vi "process_display.vi"() -> ()   [LabVIEW 2011, in "Fiberscope_library.lvlib"]
uses:
  Fiberscope_library.lvlib
  typedefs/control_process_state_cluster.ctl
  typedefs/control_process_state_enum.ctl
  typedefs/element_images_cluster.ctl
  typedefs/feedback_to_watchdog.ctl
  typedefs/feedback_from_process_enum.ctl
  typedefs/image_size_I32.ctl
  <vilib>/Analysis/NI_AALBase.lvlib
panel:
  out "Ch1 Min":u16
  out "Ch1 Max":u16
  in  "Ch1 Software gain":dbl=1.0 min=0.5 max=2.0 step=0.1
  in  "Ch1 Full range":bool
  in  "Ch1 Optimize":bool
  in  "Ch1 Color":T1(radio)
  out "Ch1 Histogram":T2(graph)
  out "Channel 1":u16[][](graph)
  in  "Ch0 Software gain":dbl=1.0 min=0.5 max=2.0 step=0.1
  out "Ch0 Histogram":T2(graph)
  in  "Ch0 Color":T1(radio)
  out "Ch0 Min":u16
  out "Ch0 Max":u16
  in  "Ch0 Full range":bool
  out "Channel 0":u16[][](graph)
  in  "Ch0 Optimize":bool
  out "Local exit":bool
  out "error out":errorcluster
  in  "error in":errorcluster
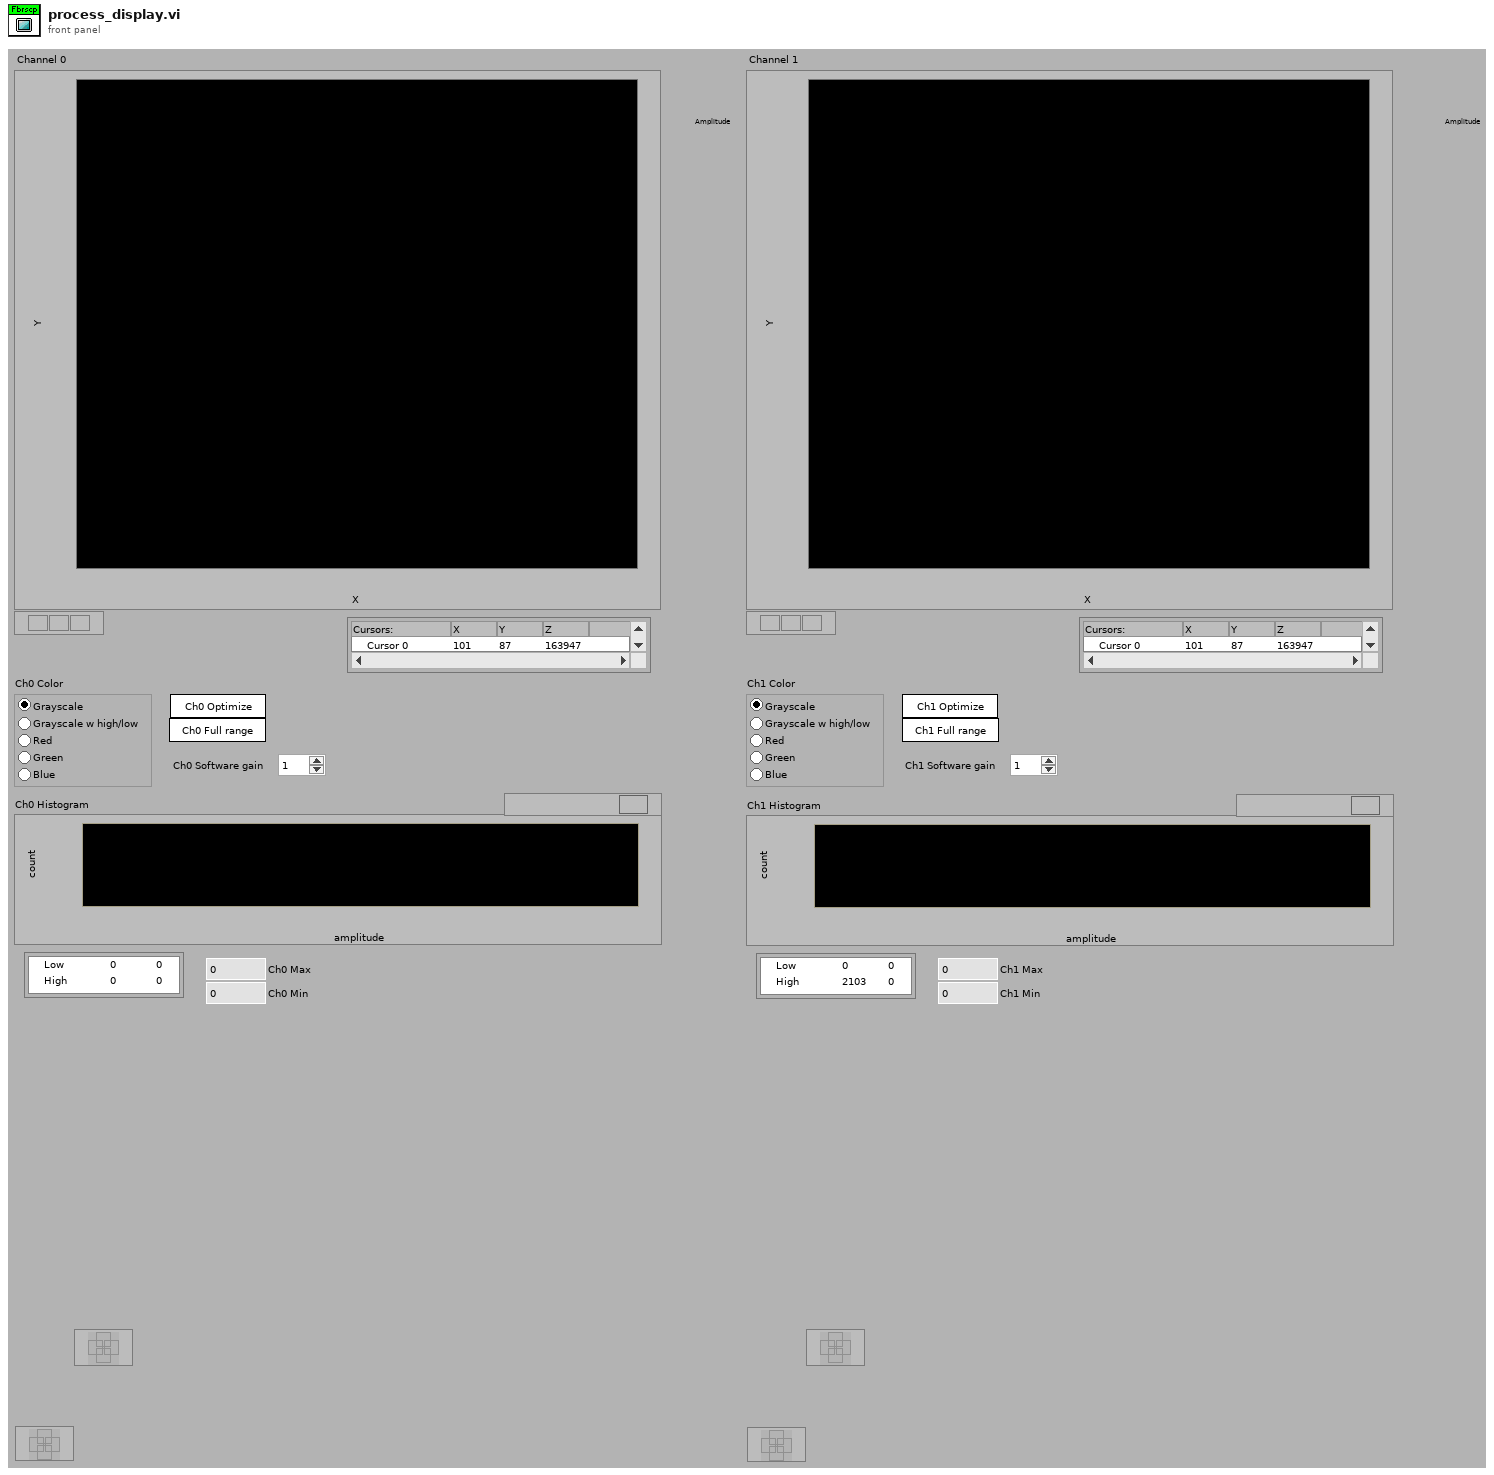
[diagram p1: front panel]
types:
  T1 = enum32{"Grayscale", "Grayscale w high/low", "Red", "Green", "Blue"}
  T2 = cluster{"X Values":dbl[], "Histogram: h(x)":i32[]}
  T3 = typedef "Fiberscope_library.lvlib/feedback_to_watchdog.ctl" = cluster{"Feedback_from_process_enum":T4, "Process_name":string}
  T4 = typedef "Fiberscope_library.lvlib/feedback_from_process_enum.ctl" = enum16{"Has_initialised", "Changed_parameters", "Has_started", "Has_stopped", "Has_quitted", "Is_running", "Has_finished", "Custom"}
  T5 = typedef "Fiberscope_library.lvlib/element_images_cluster.ctl" = cluster{"Images_array":dbl[][][], "#channels":i32, "Last element?":bool}
  T6 = typedef "Fiberscope_library.lvlib/control_process_state_cluster.ctl" = cluster{"Control_process_state_enum":T7, "variant":variant}
  T7 = typedef "Fiberscope_library.lvlib/control_process_state_enum.ctl" = enum16{"Init", "Quit", "Start", "Stop", "Change_parameters", "Running", "Finish", "Custom"}
  T8 = typedef "LVCursorListTypeDef.ctl" = cluster{"Name":string, "Color":u32, "Style":u8, "Point Style":u8, "Name Visible":bool, "Allow Drag":bool, "Cursor Mode":u32, "Plot":i32, "Index":i32, "Position":cluster{"X":dbl, "Y":dbl}, "X Scale":u32, "Y Scale":u32, "Watch Plots":i32[], "Watch All Plots":bool, "Plot Area":i32, "Label Offset":cluster{"X":dbl, "Y":dbl}}[]
  T9 = cluster{"Name":string, "Color":u32, "Style":u8, "Point Style":u8, "Name Visible":bool, "Allow Drag":bool, "Cursor Mode":u32, "Plot":i32, "Index":i32, "Position":cluster{"X":dbl, "Y":dbl}, "X Scale":u32, "Y Scale":u32, "Watch Plots":i32[], "Watch All Plots":bool, "Plot Area":i32, "Label Offset":cluster{"X":dbl, "Y":dbl}}
  T10 = cluster{"Name":string, "Color":u32, "Style":u8, "Point Style":u8, "Name Visible":bool, "Allow Drag":bool, "Cursor Mode":u32, "Plot":i32, "Index":i32, "Position":cluster{"X":dbl, "Y":dbl}, "X Scale":u32, "Y Scale":u32, "Watch Plots":i32[], "Watch All Plots":bool, "Plot Area":i32, "Label Offset":cluster{"X":dbl, "Y":dbl}}[]
  T11 = typedef "Fiberscope_library.lvlib/image_size_I32.ctl" = i32
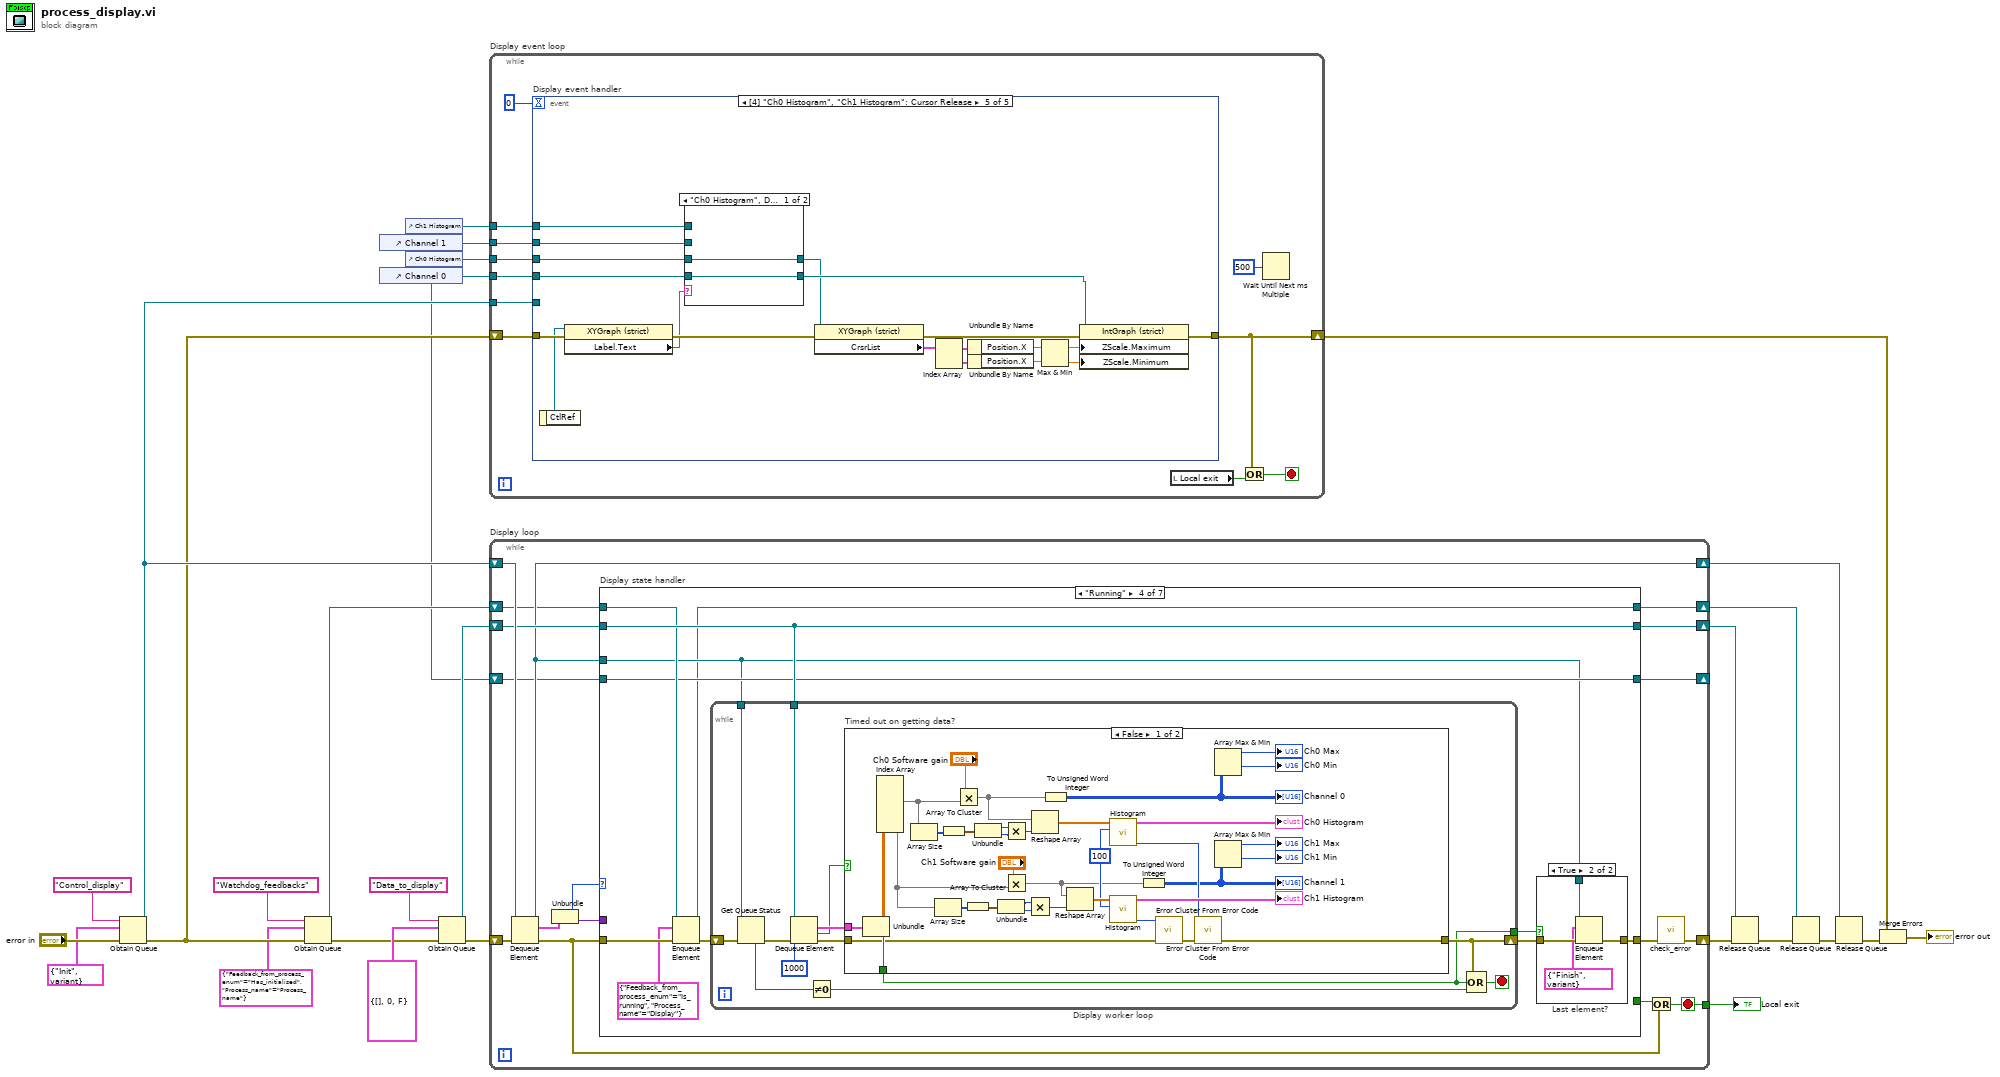
[diagram p0: block diagram]
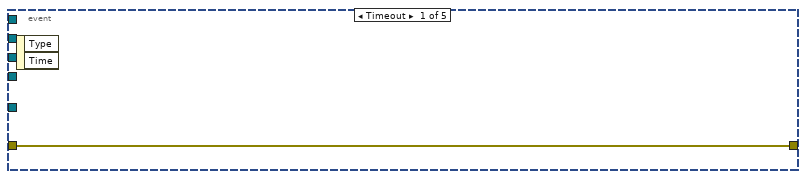
[diagram p2: hidden frame]
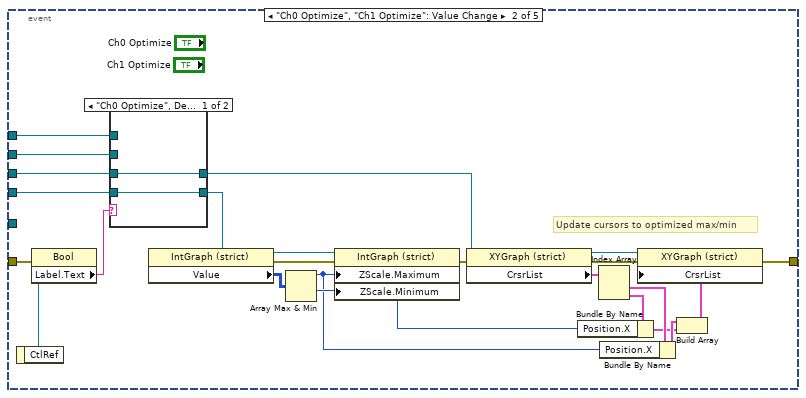
[diagram p3: hidden frame]
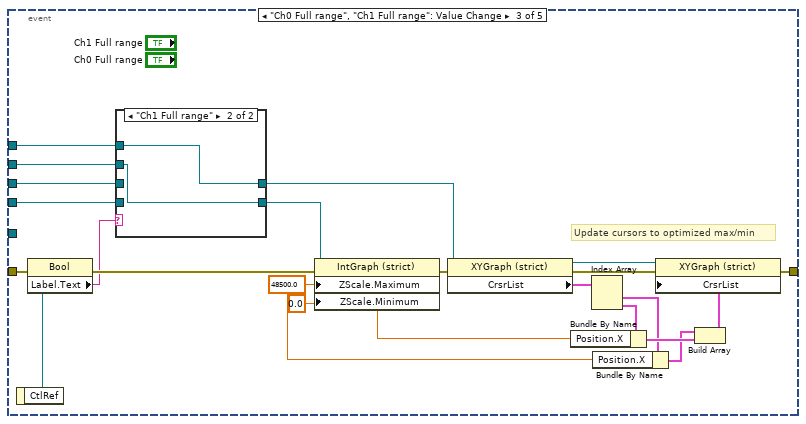
[diagram p5: hidden frame]
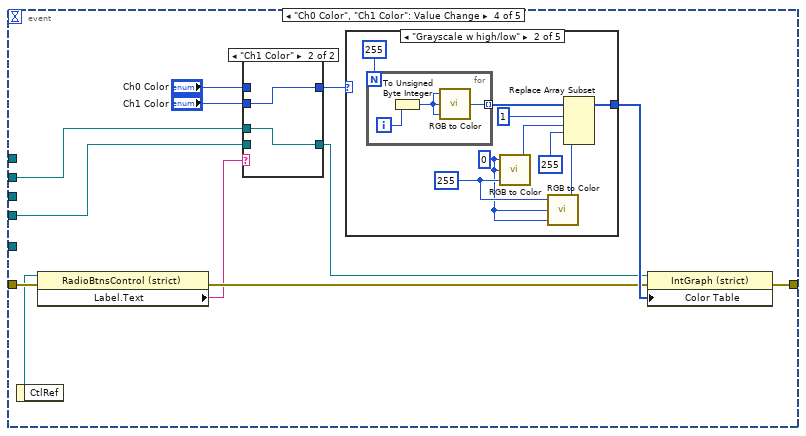
[diagram p7: hidden frame]
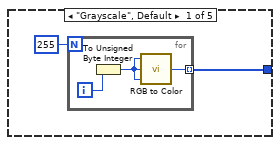
[diagram p9: hidden frame]
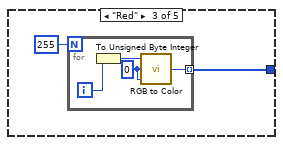
[diagram p10: hidden frame]
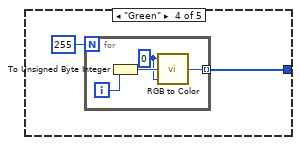
[diagram p11: hidden frame]
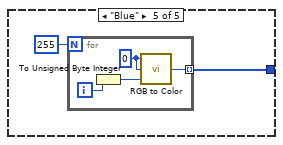
[diagram p12: hidden frame]
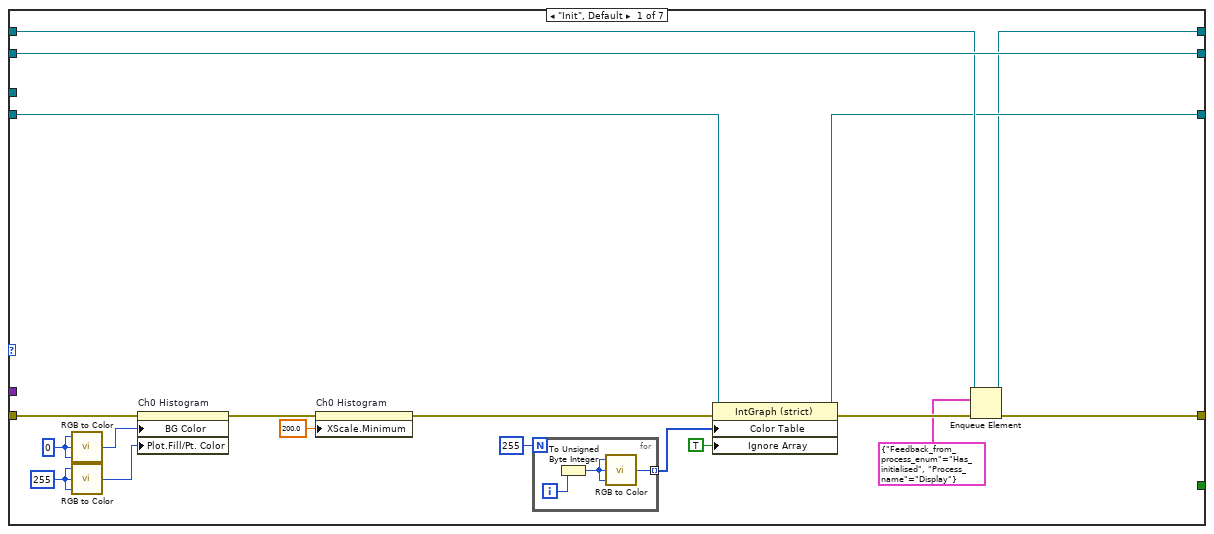
[diagram p14: hidden frame]
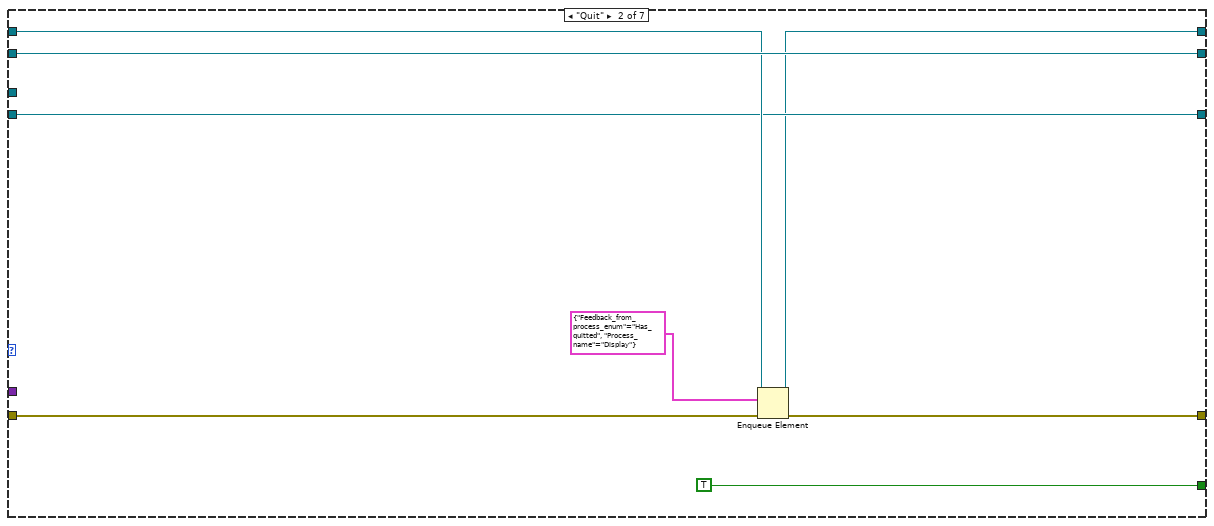
[diagram p15: hidden frame]
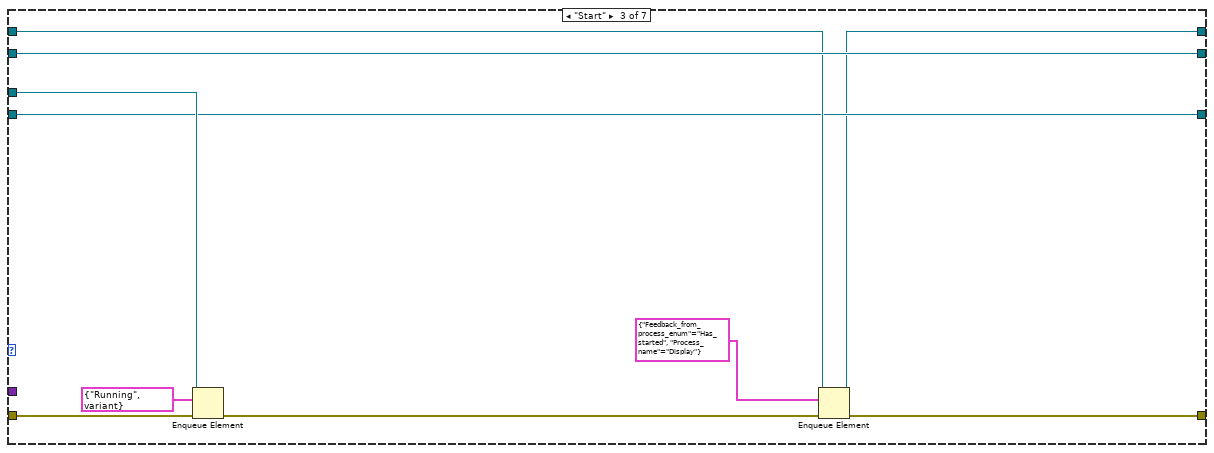
[diagram p16: hidden frame]
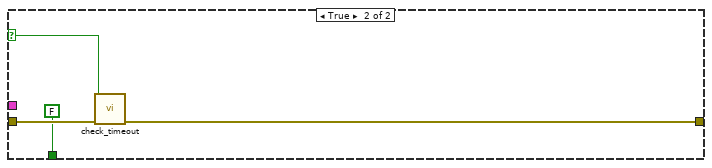
[diagram p18: hidden frame]
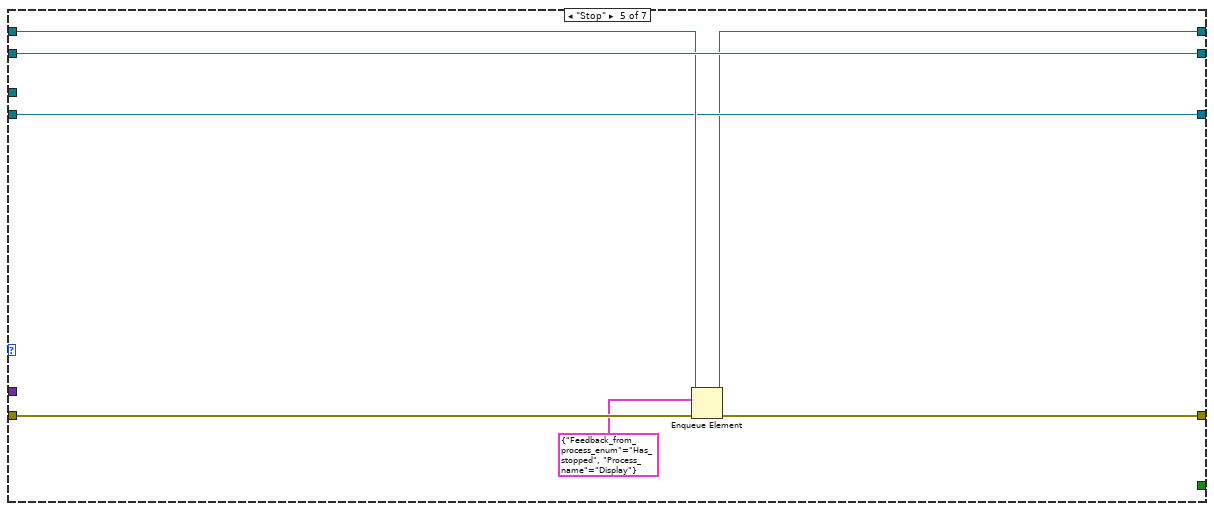
[diagram p19: hidden frame]
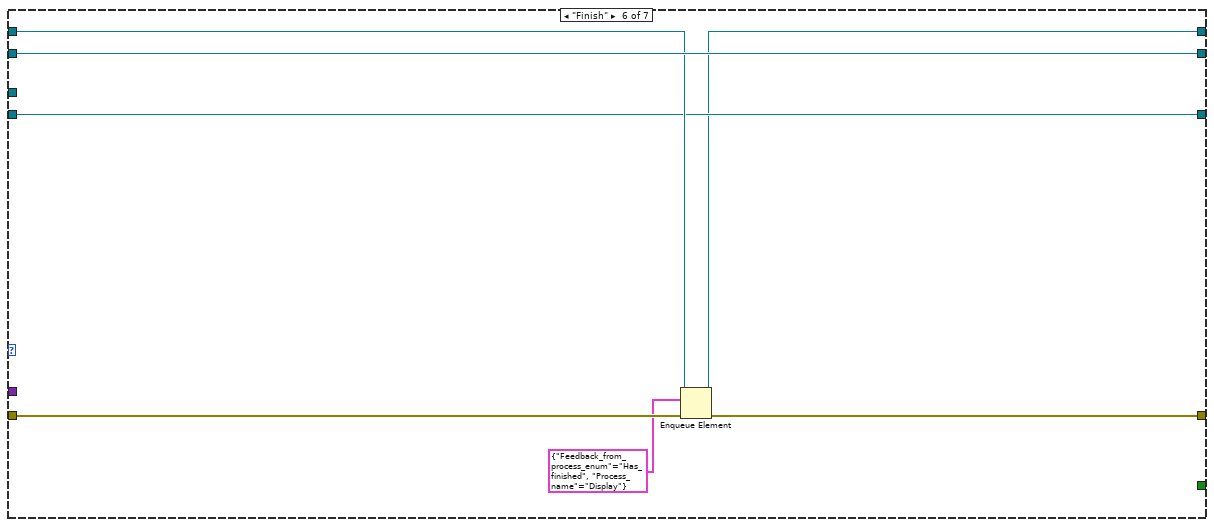
[diagram p20: hidden frame]
diagram:
  n1 = Obtain Queue(name (unnamed)="Control_display", element data type=T6 {"Control_process_state_enum"=enum."Init", "variant"=variant} ("Control_process_state_cluster"), error in (no error)="error in") -> (queue out=w16:refnum<queue>, error out=w11:errorcluster)  [unwired: 2 in, 1 out]
  n2 = Obtain Queue(name (unnamed)="Watchdog_feedbacks", element data type=T3 {"Feedback_from_process_enum"=enum."Has_initialised", "Process_name"="Process_name"}, error in (no error)=w11) -> (queue out=w9:refnum<queue>, error out=w10:errorcluster)  [unwired: 2 in, 1 out]
  n3 = control-ref of="Channel 1"() -> (w2:refnum<vi>)
  n4 = control-ref of="Channel 0"() -> (w5:refnum<vi>)
  n5 = control-ref of="Ch1 Histogram"() -> (w1:refnum<vi>)
  n6 = control-ref of="Ch0 Histogram"() -> (w4:refnum<vi>)
  n7 = Obtain Queue(name (unnamed)="Data_to_display", element data type=T5 {"Images_array"=[], "#channels"=0, "Last element?"=FALSE} ("Image out"), error in (no error)=w10) -> (queue out=w21:refnum<queue>, error out=w23:errorcluster)  [unwired: 2 in, 1 out]
  n8 = while "Display event loop" {
    tunnel: w16 -> [w37]
    shift-right: [w32] -> w14
    shift-left: w11 -> [w36]
    tunnel: w4 -> [w30]
    tunnel: w5 -> [w31]
    tunnel: w2 -> [w29]
    tunnel: w1 -> [w28]
    stop <- w33 stop-if-true
    n9 = event "Display event handler" shown="[4] \"Ch0 Histogram\", \"Ch1 Histogram\": Cursor Release" {
      selector: _ -> [_ _ _ _ _]
      dyn-events: _ -> [_ _ _ _ _]
      timeout: 0 -> [_ _ _ _ _]
      tunnel: w37 -> [_ _ _ _ _]
      tunnel: w36 -> [w39 w40 w77 w103 w148]
      tunnel: [w39 w60 w80 w105 w161] -> w32
      tunnel: w31 -> [_ w45 w71 w97 w154]
      tunnel: w30 -> [_ w46 w72 _ w153]
      tunnel: w29 -> [_ w47 w73 w96 w152]
      tunnel: w28 -> [_ w48 w74 _ w151]
      event Timeout {
        n10 = event-data() -> ()  [unwired: 1 in, 2 out]
      }
      event "Ch0 Optimize", "Ch1 Optimize": Value Change {
        # "Update cursors to optimized max/min"
        n11 = event-data() -> ("CtlRef"=w42:refnum<vi>)  [unwired: 1 in]
        n12 = property class="Bool"(reference=w42, error in=w40) -> ("Label.Text"=w41:string)  [unwired: 2 out]
        n13 = case shown="\"Ch0 Optimize\", Default" w41 {
          tunnel: w48 -> [_ w66]
          tunnel: w47 -> [_ w67]
          tunnel: w46 -> [w64 _]
          tunnel: w45 -> [w65 _]
          tunnel: [w65 w67] -> w44
          tunnel: [w64 w66] -> w43
          frame "Ch0 Optimize", Default {
          }
          frame "Ch1 Optimize" {
          }
        }
        n14 = property class="IntGraph (strict)"(reference=w44) -> (reference out=w61:refnum<vi>, error out=w63:errorcluster, "Value"=w62:u16[][])  [unwired: 1 in]
        n15 = Array Max & Min(array=w62) -> (max value=w52:u16, min value=w53:u16)  [unwired: 2 out]
        n16 = property class="IntGraph (strict)"(reference=w61, error in=w63, "ZScale.Maximum"=w52, "ZScale.Minimum"=w53) -> (error out=w59:errorcluster)  [unwired: 1 out]
        n17 = property class="XYGraph (strict)"(reference=w43, error in=w59) -> (reference out=w57:refnum<vi>, error out=w58:errorcluster, "CrsrList"=w56:T8)
        n18 = Index Array(array=w56) -> (element #1=w55:T9, element #2=w54:T9)  [unwired: 2 in]
        n19 = Bundle By Name(cluster=w54, "Position.X"=w53) -> (w50:T9)
        n20 = Bundle By Name(cluster=w55, "Position.X"=w52) -> (w51:T9)
        n21 = Build Array(w51, w50) -> (w49:T10)
        n22 = property class="XYGraph (strict)"(reference=w57, error in=w58, "CrsrList"=w49) -> (error out=w60:errorcluster)  [unwired: 1 out]
      }
      event "Ch0 Full range", "Ch1 Full range": Value Change {
        w79 = 0.0 ("Z Scale.Range:Minimum")
        w78 = 48500.0 ("Z Scale.Range:Maximum")
        # "Update cursors to optimized max/min"
        n23 = event-data() -> ("CtlRef"=w75:refnum<vi>)  [unwired: 1 in]
        n24 = property class="Bool"(reference=w75, error in=w77) -> (error out=w76:errorcluster, "Label.Text"=w70:string)  [unwired: 1 out]
        n25 = case shown="\"Ch1 Full range\"" w70 {
          tunnel: w74 -> [_ w92]
          tunnel: w73 -> [_ w93]
          tunnel: w72 -> [w90 _]
          tunnel: w71 -> [w91 _]
          tunnel: [w91 w93] -> w69
          tunnel: [w90 w92] -> w68
          frame "Ch0 Full range", Default {
          }
          frame "Ch1 Full range" {
          }
        }
        n26 = property class="IntGraph (strict)"(reference=w69, error in=w76, "ZScale.Maximum"=w78, "ZScale.Minimum"=w79) -> (error out=w81:errorcluster)  [unwired: 1 out]
        n27 = property class="XYGraph (strict)"(reference=w68, error in=w81) -> (reference out=w83:refnum<vi>, error out=w82:errorcluster, "CrsrList"=w84:T8)
        n28 = Index Array(array=w84) -> (element #1=w85:T9, element #2=w86:T9)  [unwired: 2 in]
        n29 = Bundle By Name(cluster=w86, "Position.X"=w79) -> (w88:T9)
        n30 = Bundle By Name(cluster=w85, "Position.X"=w78) -> (w87:T9)
        n31 = Build Array(w87, w88) -> (w89:T10)
        n32 = property class="XYGraph (strict)"(reference=w83, error in=w82, "CrsrList"=w89) -> (error out=w80:errorcluster)  [unwired: 1 out]
      }
      event "Ch0 Color", "Ch1 Color": Value Change {
        n33 = event-data() -> ("CtlRef"=w101:refnum<vi>)  [unwired: 1 in]
        n34 = property class="RadioBtnsControl (strict)"(reference=w101, error in=w103) -> (error out=w102:errorcluster, "Label.Text"=w94:string)  [unwired: 1 out]
        n35 = case shown="\"Ch1 Color\"" w94 {
          tunnel: "Ch0 Color" -> [w107 _]
          tunnel: "Ch1 Color" -> [_ w109]
          tunnel: [w107 w109] -> w98
          tunnel: w97 -> [w106 _]
          tunnel: w96 -> [_ w108]
          tunnel: [w106 w108] -> w95
          frame "Ch0 Color", Default {
          }
          frame "Ch1 Color" {
          }
        }
        n36 = case shown="\"Grayscale w high/low\"" w98 {
          tunnel: [w110 w115 w127 w133 w139] -> w104
          frame "Grayscale", Default {
            n37 = for {
              N: 255 -> [_]
              tunnel: [w114] -> w110 mode=indexing
              i -> [w113]
              n38 = To Unsigned Byte Integer(number=w113) -> (unsigned 8bit integer=w112:u8)
              n39 = call <vilib>:"RGB to Color.vi"("B"=w112, "G"=w112, "R"=w112) -> ("Color"=w114:u32)
            }
          }
          frame "Grayscale w high/low" {
            w116 = u8 0 ("R")
            w117 = u8 255 ("B")
            n40 = for {
              N: 255 -> [_]
              tunnel: [w126] -> w122 mode=indexing
              i -> [w125]
              n41 = To Unsigned Byte Integer(number=w125) -> (unsigned 8bit integer=w124:u8)
              n42 = call <vilib>:"RGB to Color.vi"("B"=w124, "G"=w124, "R"=w124) -> ("Color"=w126:u32)
            }
            n43 = call <vilib>:"RGB to Color.vi"("B"=w117, "G"=w116, "R"=w116) -> ("Color"=w120:u32)
            n44 = call <vilib>:"RGB to Color.vi"("B"=w116, "G"=w116, "R"=w117) -> ("Color"=w118:u32)
            n45 = Replace Array Subset(array=w122, new element #1=w120, index #1=1 ("index"), new element #2=w118, index #2=255 ("index")) -> (w115:u32[])
          }
          frame "Red" {
            n46 = for {
              N: 255 -> [_]
              tunnel: [w132] -> w127 mode=indexing
              i -> [w131]
              w129 = u8 0 ("G")
              n47 = To Unsigned Byte Integer(number=w131) -> (unsigned 8bit integer=w130:u8)
              n48 = call <vilib>:"RGB to Color.vi"("B"=w129, "G"=w129, "R"=w130) -> ("Color"=w132:u32)
            }
          }
          frame "Green" {
            n49 = for {
              N: 255 -> [_]
              tunnel: [w138] -> w133 mode=indexing
              i -> [w137]
              w135 = u8 0 ("R")
              n50 = To Unsigned Byte Integer(number=w137) -> (unsigned 8bit integer=w136:u8)
              n51 = call <vilib>:"RGB to Color.vi"("B"=w135, "G"=w136, "R"=w135) -> ("Color"=w138:u32)
            }
          }
          frame "Blue" {
            n52 = for {
              N: 255 -> [_]
              tunnel: [w144] -> w139 mode=indexing
              i -> [w143]
              w141 = u8 0 ("R")
              n53 = To Unsigned Byte Integer(number=w143) -> (unsigned 8bit integer=w142:u8)
              n54 = call <vilib>:"RGB to Color.vi"("B"=w142, "G"=w141, "R"=w141) -> ("Color"=w144:u32)
            }
          }
        }
        n55 = property class="IntGraph (strict)"(reference=w95, error in=w102, "Color Table"=w104) -> (error out=w105:errorcluster)  [unwired: 1 out]
      }
      event "Ch0 Histogram", "Ch1 Histogram": Cursor Release {
        n56 = event-data() -> ("CtlRef"=w146:refnum<vi>)  [unwired: 1 in]
        n57 = property class="XYGraph (strict)"(reference=w146, error in=w148) -> (error out=w147:errorcluster, "Label.Text"=w145:string)  [unwired: 1 out]
        n58 = case shown="\"Ch0 Histogram\", Default" w145 {
          tunnel: w151 -> [_ w166]
          tunnel: w152 -> [_ w167]
          tunnel: w153 -> [w164 _]
          tunnel: w154 -> [w165 _]
          tunnel: [w165 w167] -> w150
          tunnel: [w164 w166] -> w149
          frame "Ch0 Histogram", Default {
          }
          frame "Ch1 Histogram" {
          }
        }
        n59 = property class="XYGraph (strict)"(reference=w149, error in=w147) -> (error out=w162:errorcluster, "CrsrList"=w163:T8)  [unwired: 1 out]
        n60 = Index Array(array=w163) -> (element #1=w160:T9, element #2=w159:T9)  [unwired: 2 in]
        n61 = Unbundle By Name(w160) -> ("Position.X"=w158:dbl)
        n62 = Unbundle By Name(w159) -> ("Position.X"=w157:dbl)
        n63 = Max & Min(x=w158, y=w157) -> (max(x,y)=w156:dbl, min(x,y)=w155:dbl)
        n64 = property class="IntGraph (strict)"(reference=w150, error in=w162, "ZScale.Maximum"=w156, "ZScale.Minimum"=w155) -> (error out=w161:errorcluster)  [unwired: 1 out]
      }
    }
    n65 = local read "Local exit"() -> (w34:bool)
    n66 = Or(x=w32, y=w34) -> (x .or. y?=w33:bool)
    n67 = Wait Until Next ms Multiple(millisecond multiple=u32 500) -> ()  [unwired: 1 out]
  }
  n68 = while "Display loop" {
    shift-right: [w178] -> w20
    shift-left: w23 -> [w184]
    shift-right: [w175] -> w25
    shift-left: w16 -> [w183]
    shift-right: [w176] -> w19
    shift-left: w21 -> [w177]
    tunnel: [w174] -> w17
    shift-right: [w168] -> w6
    shift-left: w9 -> [w171]
    shift-right: [w169] -> _
    shift-left: w5 -> [w170]
    stop <- w174 stop-if-true
    n69 = Dequeue Element(queue=w183, error in (no error)=w184) -> (queue out=w175:refnum<queue>, element=w182:T6, error out=w172:errorcluster)  [unwired: 1 in, 1 out]
    n70 = Unbundle(w182) -> ("Control_process_state_enum"=w180:T7, "variant"=w181:variant)
    n71 = case "Display state handler" shown="\"Running\"" w180 {
      tunnel: w172 -> [w190 w212 w221 w234 w298 w305 w325]
      tunnel: [w202 w211 w223 w229 w297 w304 w319] -> w179
      tunnel: w181 -> [_ _ _ _ _ _ w324]
      tunnel: w177 -> [w203 w214 w224 w235 w299 w306 w326]
      tunnel: [w203 w214 w224 w235 w299 w306 w326] -> w176
      tunnel: w175 -> [_ _ w219 w228 _ _ _]
      tunnel: [_ TRUE _ _ _ _ _] -> w173
      tunnel: w171 -> [w201 w210 w222 w232 w296 w303 w318]
      tunnel: w170 -> [w199 w209 w218 w231 w295 w302 w317]
      tunnel: [w198 w209 w218 w231 w295 w302 w317] -> w169
      tunnel: [w189 w208 w216 w226 w294 w301 w314] -> w168
      frame "Init", Default {
        w193 = u8 0 ("R")
        w194 = u8 255 ("R")
        n72 = call <vilib>:"RGB to Color.vi"("B"=w193, "G"=w193, "R"=w193) -> ("Color"=w192:u32)
        n73 = call <vilib>:"RGB to Color.vi"("B"=w194, "G"=w194, "R"=w194) -> ("Color"=w191:u32)
        n74 = property on="Ch0 Histogram" class="XYGraph (strict)"(error in=w190, "BG Color"=w192, "Plot.Fill/Pt. Color"=w191) -> (error out=w187:errorcluster)  [unwired: 1 in, 1 out]
        n75 = property on="Ch0 Histogram" class="XYGraph (strict)"(error in=w187, "XScale.Minimum"=200.0 ("X Scale.Range:Minimum")) -> (error out=w186:errorcluster)  [unwired: 1 in, 1 out]
        n76 = for {
          N: 255 -> [_]
          tunnel: [w206] -> w195 mode=indexing
          i -> [w205]
          n77 = To Unsigned Byte Integer(number=w205) -> (unsigned 8bit integer=w204:u8)
          n78 = call <vilib>:"RGB to Color.vi"("B"=w204, "G"=w204, "R"=w204) -> ("Color"=w206:u32)
        }
        n79 = property class="IntGraph (strict)"(reference=w199, error in=w186, "Color Table"=w195, "Ignore Array"=TRUE) -> (reference out=w198:refnum<vi>, error out=w200:errorcluster)
        n80 = Enqueue Element(queue=w201, element=T3 {"Feedback_from_process_enum"=enum."Has_initialised", "Process_name"="Display"}, error in (no error)=w200) -> (queue out=w189:refnum<queue>, error out=w202:errorcluster)  [unwired: 1 in, 1 out]
      }
      frame "Quit" {
        n81 = Enqueue Element(queue=w210, element=T3 {"Feedback_from_process_enum"=enum."Has_quitted", "Process_name"="Display"}, error in (no error)=w212) -> (queue out=w208:refnum<queue>, error out=w211:errorcluster)  [unwired: 1 in, 1 out]
      }
      frame "Start" {
        n82 = Enqueue Element(queue=w219, element=T6 {"Control_process_state_enum"=enum."Running", "variant"=variant} ("Control_process_state_cluster"), error in (no error)=w221) -> (error out=w220:errorcluster)  [unwired: 1 in, 2 out]
        n83 = Enqueue Element(queue=w222, element=T3 {"Feedback_from_process_enum"=enum."Has_started", "Process_name"="Display"}, error in (no error)=w220) -> (queue out=w216:refnum<queue>, error out=w223:errorcluster)  [unwired: 1 in, 1 out]
      }
      frame "Running" {
        n84 = Enqueue Element(queue=w232, element=T3 {"Feedback_from_process_enum"=enum."Is_running", "Process_name"="Display"}, error in (no error)=w234) -> (queue out=w226:refnum<queue>, error out=w233:errorcluster)  [unwired: 1 in, 1 out]
        n85 = while "Display worker loop" {
          tunnel: w228 -> [w252]
          tunnel: w235 -> [w249]
          shift-right: [w242] -> w230
          shift-left: w233 -> [w253]
          tunnel: [w241] -> w227
          stop <- w247 stop-if-true
          n86 = Get Queue Status(queue=w252, error in (no error)=w253) -> (error out=w250:errorcluster, # elements in queue=w251:i32)  [unwired: 1 in, 6 out]
          n87 = Dequeue Element(queue=w249, timeout in ms (-1)=1000, error in (no error)=w250) -> (element=w246:T5, timed out?=w243:bool, error out=w245:errorcluster)  [unwired: 1 out]
          n88 = Not Equal To 0?(x=w251) -> (x != 0?=w248:bool)
          n89 = case "Timed out on getting data?" shown="False" w243 {
            selector: w243 -> [_ w290]
            tunnel: w246 -> [w286 _]
            tunnel: w245 -> [w282 w292]
            tunnel: [w261 w291] -> w242
            tunnel: [w284 FALSE ("Last element?")] -> w241
            frame False {
              w263 = 100 ("intervals")
              n90 = Unbundle(w286) -> ("Images_array"=w285:dbl[][][], "Last element?"=w284:bool)  [unwired: 1 out]
              n91 = Index Array(array=w285) -> (element #1=w278:dbl[][], element #2=w266:dbl[][])  [unwired: 6 in]
              n92 = Array Size(array=w278) -> (size(s)=w277:i32[])
              n93 = Array Size(array=w266) -> (size(s)=w271:i32[])
              n94 = Array To Cluster(array=w277) -> (cluster=w276:cluster{"[0]":i32, "[1]":i32})
              n95 = Multiply(x="Ch0 Software gain", y=w278) -> (x*y=w279:dbl[][])
              n96 = Array To Cluster(array=w271) -> (cluster=w270:cluster{"[0]":i32, "[1]":i32})
              n97 = Unbundle(w276) -> ("[0]"=w275:i32, "[1]"=w274:i32)
              n98 = Unbundle(w270) -> ("[0]"=w268:i32, "[1]"=w267:i32)
              n99 = Multiply(x=w275, y=w274) -> (x*y=w273:i32)
              n100 = Multiply(x="Ch1 Software gain", y=w266) -> (x*y=w257:dbl[][])
              n101 = Multiply(x=w268, y=w267) -> (x*y=w265:i32)
              n102 = Reshape Array(w279, w273) -> (w283:dbl[])
              n103 = To Unsigned Word Integer(number=w279) -> (unsigned 16bit integer=w272:u16[][])
              "Channel 0" <- w272
              n104 = Reshape Array(w257, w265) -> (w264:dbl[])
              n105 = call <vilib>:"Histogram.vi"("intervals"=w263, "X"=w283) -> ("error"=w258:i32, "Histogram Graph"=→"Ch0 Histogram":T2)  [unwired: 6 in, 2 out]
              n106 = call <vilib>:"Histogram.vi"("intervals"=w263, "X"=w264) -> ("error"=w260:i32, "Histogram Graph"=→"Ch1 Histogram":T2)  [unwired: 6 in, 2 out]
              n107 = To Unsigned Word Integer(number=w257) -> (unsigned 16bit integer=w256:u16[][])
              "Channel 1" <- w256
              n108 = call <vilib>:"Error Cluster From Error Code.vi"("error in (no error)"=w282, "error code (0)"=w260) -> ("error out"=w262:errorcluster)  [unwired: 7 in]
              n109 = call <vilib>:"Error Cluster From Error Code.vi"("error in (no error)"=w262, "error code (0)"=w258) -> ("error out"=w261:errorcluster)  [unwired: 7 in]
              n110 = Array Max & Min(array=w272) -> (max value=→"Ch0 Max":u16, min value=→"Ch0 Min":u16)  [unwired: 2 out]
              n111 = Array Max & Min(array=w256) -> (max value=→"Ch1 Max":u16, min value=→"Ch1 Min":u16)  [unwired: 2 out]
            }
            frame True {
              n112 = call "check_timeout.vi"("error in"=w292, "Timeout?"=w290) -> ("error out"=w291:errorcluster)  [unwired: 9 in]
            }
          }
          n113 = Compound Arithmetic op=OR(w242, w241, w248) -> (w247:bool)
        }
        n114 = case "Last element?" shown="True" w227 {
          tunnel: w230 -> [w236 w240]
          tunnel: [w236 w239] -> w229
          tunnel: w228 -> [_ w238]
          frame False {
          }
          frame True {
            n115 = Enqueue Element(queue=w238, element=T6 {"Control_process_state_enum"=enum."Finish", "variant"=variant} ("Control_process_state_cluster"), error in (no error)=w240) -> (error out=w239:errorcluster)  [unwired: 1 in, 2 out]
          }
        }
      }
      frame "Stop" {
        n116 = Enqueue Element(queue=w296, element=T3 {"Feedback_from_process_enum"=enum."Has_stopped", "Process_name"="Display"}, error in (no error)=w298) -> (queue out=w294:refnum<queue>, error out=w297:errorcluster)  [unwired: 1 in, 1 out]
      }
      frame "Finish" {
        n117 = Enqueue Element(queue=w303, element=T3 {"Feedback_from_process_enum"=enum."Has_finished", "Process_name"="Display"}, error in (no error)=w305) -> (queue out=w301:refnum<queue>, error out=w304:errorcluster)  [unwired: 1 in, 1 out]
      }
      frame "Change_parameters" {
        w316 = T11 128 items=["128x128 px"=128, "256x256 px"=256, "512x512 px"=512] ("Image size")
        n118 = Variant To Data(error in=w325, type=w316, Variant=w324) -> (data=w315:T11, error out=w322:errorcluster)
        n119 = To Double Precision Float(number=w315) -> (double precision float=w307:dbl)
        n120 = control-ref of="Channel 0"() -> (w320:refnum<vi>)
        n121 = property class="IntGraph (strict)"(reference=w320, error in=w322, "XScale.Maximum"=w307) -> (reference out=w321:refnum<vi>, error out=w323:errorcluster)
        n122 = property class="IntGraph (strict)"(reference=w321, error in=w323, "YScale.Maximum"=w307) -> (error out=w310:errorcluster)  [unwired: 1 out]
        n123 = control-ref of="Channel 1"() -> (w308:refnum<vi>)
        n124 = property class="IntGraph (strict)"(reference=w308, error in=w310, "XScale.Maximum"=w307) -> (reference out=w311:refnum<vi>, error out=w312:errorcluster)
        n125 = property class="IntGraph (strict)"(reference=w311, error in=w312, "YScale.Maximum"=w307) -> (error out=w309:errorcluster)  [unwired: 1 out]
        n126 = Enqueue Element(queue=w318, element=T3 {"Feedback_from_process_enum"=enum."Changed_parameters", "Process_name"="Display"}, error in (no error)=w309) -> (queue out=w314:refnum<queue>, error out=w319:errorcluster)  [unwired: 1 in, 1 out]
      }
    }
    n127 = Or(x=w173, y=w172) -> (x .or. y?=w174:bool)
    n128 = call "check_error.vi"("error in"=w179) -> ("error out"=w178:errorcluster)  [unwired: 10 in]
  }
  "Local exit" <- w17
  n129 = Release Queue(queue=w19, error in (no error)=w20) -> (error out=w8:errorcluster)  [unwired: 1 in, 2 out]
  n130 = Release Queue(queue=w6, error in (no error)=w8) -> (error out=w7:errorcluster)  [unwired: 1 in, 2 out]
  n131 = Release Queue(queue=w25, error in (no error)=w7) -> (error out=w15:errorcluster)  [unwired: 1 in, 2 out]
  n132 = Merge Errors(w14, w15) -> (→"error out":errorcluster)
